vi "get_point_line_distance.vi"(8 "y":dbl, 9 "x":dbl, 10 "intercept":dbl, 11 "gradient":dbl) -> (2 "distance":dbl)   [LabVIEW 2017]
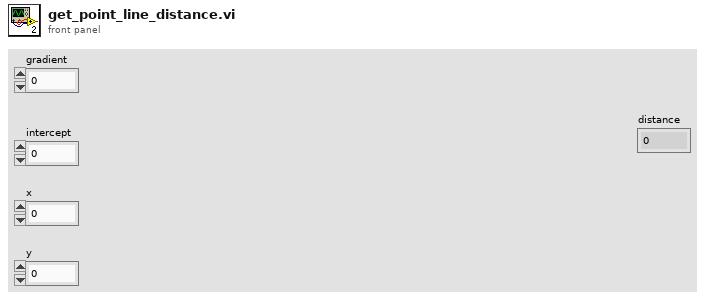
[diagram p1: front panel]
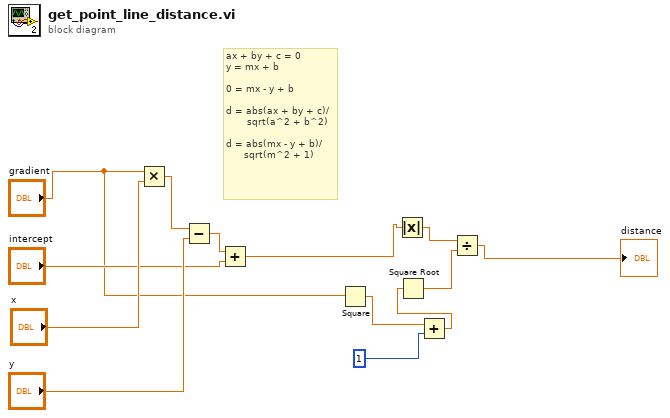
[diagram p0: block diagram]
diagram:
  # "ax + by + c = 0\ny = mx + b\n\n0 = mx - y + b\n\nd = abs(ax + by + c)/\n       sqrt(a^2 + b^2)\n\nd = abs(mx - y + b)/\n      sqrt(m^2 + 1)"
  n1 = Multiply(x="gradient", y="x") -> (x*y=w12:dbl)
  n2 = Subtract(x=w12, y="y") -> (x-y=w10:dbl)
  n3 = Add(x=w10, y="intercept") -> (x+y=w8:dbl)
  n4 = Square(x="gradient") -> (x^2=w3:dbl)
  n5 = Absolute Value(x=w8) -> (abs(x)=w7:dbl)
  n6 = Add(x=w3, y=1) -> (x+y=w1:dbl)
  n7 = Square Root(x=w1) -> (sqrt(x)=w6:dbl)
  n8 = Divide(x=w7, y=w6) -> (x/y=→"distance":dbl)
